vi "Create.vi"(8 "error in (no error)":errorcluster, 10 "Data":dbl) -> (0 "error out":errorcluster, 3 "Enqueue Data Msg out":refnum<class "Enqueue Data Msg.lvclass">)   [LabVIEW 2020, in "Scratchpad.lvlib" / "Test 1.lvlib" / "Enqueue Data Msg.lvclass"]
uses:
  Enqueue Data Msg.lvclass
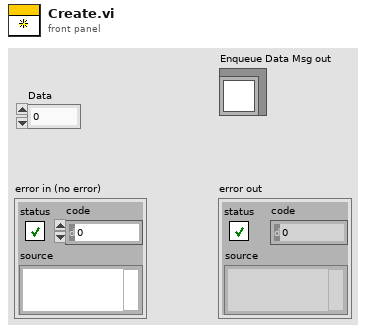
[diagram p1: front panel]
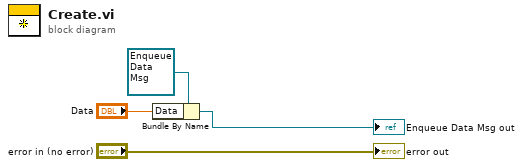
[diagram p0: block diagram]
diagram:
  n1 = Bundle By Name(cluster=refnum<class "Enqueue Data Msg.lvclass"> refnum ("Enqueue Data Msg in"), "Data"="Data") -> (→"Enqueue Data Msg out":refnum<class "Enqueue Data Msg.lvclass">)
  "error out" <- "error in (no error)"
